vi "Write To Lights.vi"   [LabVIEW 2014]
uses:
  Common Code/Utilities/TimeManager.vi
  Common Code/Change Detect.vi
  Common Code/Change Detect Boolean.vi
  Robot Global Data.vi
types:
  T1 = typedef "Elevator Status.ctl" = cluster{"Height":dbl, "Enc Value":dbl, "Limit Override":bool, "Mode":T2, "High IR":bool, "Motor Out":dbl, "Ping Detect":bool, "Auto Elevator Indicators":T3, "Master Current":dbl, "Slave Current":dbl, "High Current":bool, "Current Tripped":bool, "Top Limit":bool, "Bottom Limit":bool, "Eject Piston":bool, "Stabilizer":bool, "Finger":bool, "Finger Height":dbl, "Finger Raw":dbl, "Finger at Bottom":bool}
  T2 = typedef "Elevator Mode.ctl" = enum16{"Manual", "Safe", "Auto"}
  T3 = typedef "Auto Elevator Indicators.ctl" = cluster{"Target Out":dbl, "Storing Trashcan?":bool, "State":T4, "In Range":bool, "Store Can Command":bool, "HP Load":bool}
  T4 = typedef "Elevator State.ctl" = enum16{"Idle", "Goto Load Position", "Wait for Load", "Load Drop", "Load Lift", "Drop Stack", "Goto Eject Position", "Eject ", "Raise Trashcan", "Open Stabilizer", "Untip Drop", "Untip Wait", "Untip Lift", "Abort Load", "HP Load Wait", "HP Load Drop", "HP Load Lift", "HP Load Abort", "Close Stabilizer", "HP Load Unfinish", "HP Load Score", "HP Load Finish", "HP Goto Finish Down", "HP Goto Finish Up", "Full"}
  T5 = typedef "WPI_DriverStationRobotMode2.ctl" = enum16{"Autonomous Disabled", "Autonomous Enabled", "Teleop Disabled", "Teleop Enabled", "Disconnected", "Finish", "Test Disabled", "Test Enabled", "Emergency Stopped"}
  T6 = typedef "WPI_DriverStationAllianceInfo.ctl" = enum16{"Red", "Blue", "Invalid"}
  T7 = typedef "Dashboard Control Data.ctl" = cluster{"Cam Exposure":dbl, "Go to angle":dbl, "Steer PID Gains":cluster{"proportional gain (Kc)":dbl, "integral time (Ti, min)":dbl, "derivative time (Td, min)":dbl}, "Steer PID output Range":cluster{"output high":dbl, "output low":dbl}, "Pressure m \nValue":dbl, "Pressure b \nValue":dbl, "Roller Command Cluster ":T8, "Elevator":T9, "Encoder Control":T11, "Auton Settings":cluster{"Drive Dist Window Size":dbl}, "Drivetrain Settings":T12, "Lance":T13}
  T8 = typedef "Roller Control.ctl" = cluster{"Intake Speed":dbl, "Turn In Speed":dbl, "Unload Speed":dbl, "Turn Out Speed":dbl, "Ping Align Tolerance":dbl, "Tote Range Threshold":dbl, "Right Pot 0":dbl, "Pot Threshold":dbl, "Left Pot 0":dbl, "Right Pot Scale":dbl, "Left Pot Scale":dbl, "Min Elevator Height":dbl, "Eject Time":dbl, "Eject US Threshold":dbl, "Anti-Twitch Time":u32, "Ping Caring Threshold":dbl, "Pot Diff Threshold":dbl, "Pinch Sustain":u32, "Absorb Give Up Threshold":dbl, "Untip In Threshold":dbl, "Untip Grab Range":dbl, "Ultrasonic Hold Time":u32, "Landscape Absorb Time":u32, "Pot Use Wait Time":u32, "Can Turn Stop Range":dbl, "HP Load Speed":dbl, "Stick Multiplier":dbl}
  T9 = typedef "Elevator DB Control.ctl" = cluster{"PID Output Range":cluster{"output high":dbl, "output low":dbl}, "PID gains":cluster{"proportional gain (Kc)":dbl, "integral time (Ti, min)":dbl, "derivative time (Td, min)":dbl}, "Height Tolerance":sgl, " Encoder Constant":dbl, "Eject Time":sgl, "Zeroing Speed":sgl, "Presets":T10, "Ping Detect Threshold":sgl, "Trashcan Detect Threshold":sgl, "Zero Filter Time":dbl, "Stabilizer Open Time":dbl, "Zero Creep Speed":dbl, "Max Current":dbl, "Current Trip Time":dbl, "Abort Pitch":dbl, "Finger m":dbl, "Finger b":dbl, "Finger max ":dbl, "Finger Stabilizer":dbl, "Finger Store":dbl, "Finger Stop Store":dbl, "Stabilizer Close Time":dbl, "Finger min":dbl, "Unstick gain":dbl, "Full Detect Max":dbl}
  T10 = typedef "Elevator Presets.ctl" = cluster{"Pickup 2 w/ Tote":sgl, "Pickup 2 w/ Trashcan":sgl, "Pickup 3 w/ Tote":sgl, "Pickup 3 w/ Trashcan":sgl, "Bottom":sgl, "Pickup 1 w/ Tote":sgl, "Pickup Trashcan":sgl, "Pickup 1 w/ Trashcan":sgl, "Eject":sgl, "Hold Low":sgl, "Step add height":sgl, "Untip Lift":dbl, "Drop Stack":dbl, "HP Load Hold":dbl, "HP Load Drop":dbl, "HP Load Hold Can":dbl, "Store can max":dbl, "HP Drag Score":dbl, "HP Drag Finish":dbl, "Finger trashcan avoid":dbl, "Full":dbl}
  T11 = typedef "Encoder Control.ctl" = cluster{"Left Tick Constant":dbl, "Right Tick Constant":dbl, "Center Tick Constant":dbl, "Reset?":bool, "Y Dist":cluster{"PID gains":cluster{"proportional gain (Kc)":dbl, "integral time (Ti, min)":dbl, "derivative time (Td, min)":dbl}}, "X Dist":cluster{"PID gains":cluster{"proportional gain (Kc)":dbl, "integral time (Ti, min)":dbl, "derivative time (Td, min)":dbl}}, "Y Stop Thresh":dbl, "Y Stop Speed":dbl, "X Stop Thresh":dbl, "X Stop Speed":dbl}
  T12 = typedef "Drivetrain Settings.ctl" = cluster{"Gyro Tolerance":sgl, "Strafe Correct max steer":sgl, "Strafe Timer Wait":sgl, "Throttle Ramp (ms)":sgl, "Strafe Ramp (ms)":sgl, "Angular rate compensation":bool, "Throttle to Rate Scale":sgl, "Rate compensation gain":sgl, "Creep Steer":sgl, "Creep Throttle":sgl}
  T13 = typedef "Pike DB Controls.ctl" = cluster{"Down Speed":dbl, "Up Speed":dbl, "Max Down Time":dbl, "Max Up Time":dbl, "Current Limit":dbl}
  T14 = typedef "WPI_AOChannelDevRef.ctl" = cluster{"DevStatus":errorcluster, "Controller":T15, "AO Channel":T16}
  T15 = typedef "FPGA_TypedefAnalogModule.ctl" = enum16{"Controller 1"}
  T16 = typedef "WPI_AnalogOutputChannel.ctl" = enum8{"AO MXP 0", "AO MXP 1", "Invalid"}
  T17 = typedef "WPI_DigitalOutputDevRef.ctl" = cluster{"Controller":T18, "DIO Channel":T19, "DevStatus":errorcluster}
  T18 = typedef "FPGA_TypedefDigitalModule.ctl" = enum16{"Controller 1"}
  T19 = typedef "FPGA_DIOChannel.ctl" = enum8{"DIO 0", "DIO 1", "DIO 2", "DIO 3", "DIO 4", "DIO 5", "DIO 6", "DIO 7", "DIO 8", "DIO 9", "DIO MXP 0", "DIO MXP 1", "DIO MXP 2", "DIO MXP 3", "DIO MXP 4", "DIO MXP 5", "DIO MXP 6", "DIO MXP 7", "DIO MXP 8", "DIO MXP 9", "DIO MXP 10", "DIO MXP 11", "DIO MXP 12", "DIO MXP 13", "DIO MXP 14", "DIO MXP 15", "Invalid"}
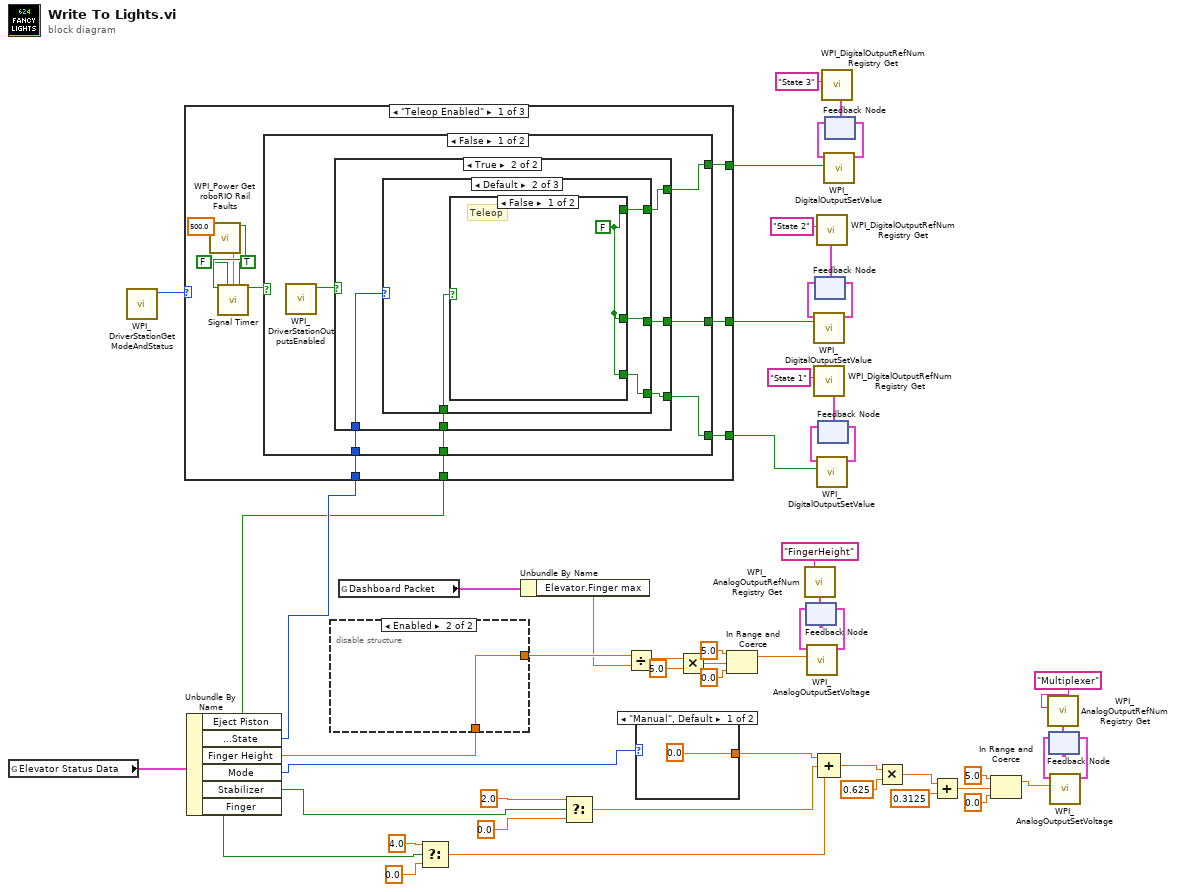
[diagram p0: block diagram]
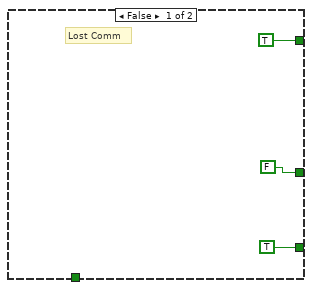
[diagram p2: hidden frame]
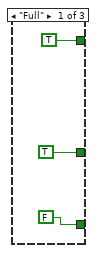
[diagram p3: hidden frame]
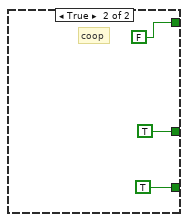
[diagram p4: hidden frame]
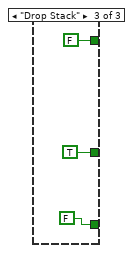
[diagram p5: hidden frame]
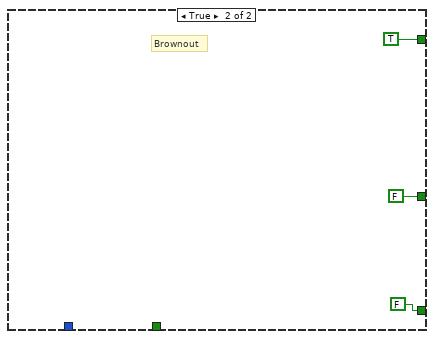
[diagram p6: hidden frame]
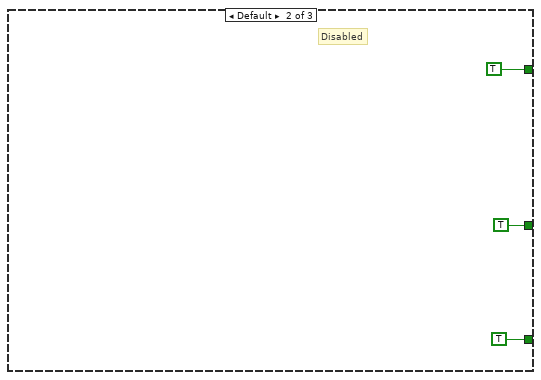
[diagram p7: hidden frame]
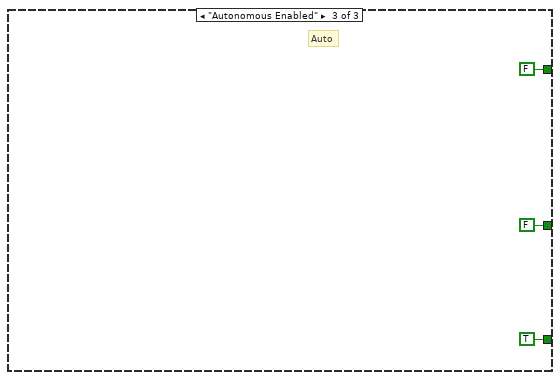
[diagram p8: hidden frame]
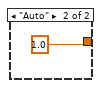
[diagram p9: hidden frame]
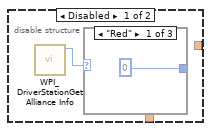
[diagram p10: hidden frame]
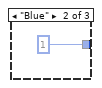
[diagram p11: hidden frame]
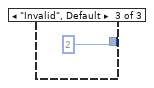
[diagram p12: hidden frame]
diagram:
  n1 = global read "Robot Global Data.vi" "Elevator Status Data"() -> (w43:T1)
  n2 = call <vilib>:"WPI_DriverStationGetModeAndStatus.vi"() -> ("Robot Mode"=w6:T5)  [unwired: 10 in, 1 out]
  n3 = Unbundle By Name(w43) -> ("Eject Piston"=w1:bool, "Auto Elevator Indicators.State"=w2:T4, "Finger Height"=w40:dbl, "Mode"=w38:T2, "Stabilizer"=w39:bool, "Finger"=w35:bool)
  n4 = case shown="\"Teleop Enabled\"" w6 {
    tunnel: [w65 TRUE FALSE] -> w5
    tunnel: [w64 TRUE FALSE] -> w4
    tunnel: [w63 TRUE TRUE] -> w3
    tunnel: w2 -> [w62 _ _]
    tunnel: w1 -> [w61 _ _]
    frame "Teleop Enabled" {
      n5 = call <vilib>:"WPI_Power Get roboRIO Rail Faults.vi"() -> ("Input Voltage Brown Out"=w60:bool)  [unwired: 11 in, 4 out]
      n6 = call "Signal Timer.vi"("Input"=w60, "Edge"=FALSE, "Interval"=500.0, "Pull"=TRUE) -> ("Filtered Output"=w56:bool)  [unwired: 11 in]
      n7 = case shown="False" w56 {
        tunnel: [w68 TRUE] -> w65
        tunnel: [w69 FALSE] -> w64
        tunnel: [w70 FALSE] -> w63
        tunnel: w62 -> [w67 _]
        tunnel: w61 -> [w66 _]
        frame False {
          n8 = call <vilib>:"WPI_DriverStationOutputsEnabled.vi"() -> ("OutputsEnabled?"=w71:bool)  [unwired: 10 in, 1 out]
          n9 = case shown="True" w71 {
            tunnel: [TRUE w76] -> w70
            tunnel: [FALSE w77] -> w69
            tunnel: [TRUE w78] -> w68
            tunnel: w67 -> [_ w79]
            tunnel: w66 -> [_ w75]
            frame False {
              # "Lost Comm"
            }
            frame True {
              n10 = case shown="Default" w79 {
                tunnel: [TRUE w86 FALSE] -> w78
                tunnel: [TRUE w84 TRUE] -> w77
                tunnel: [FALSE w85 FALSE] -> w76
                tunnel: w75 -> [_ w83 _]
                frame "Full" {
                }
                frame Default {
                  n11 = case shown="False" w83 {
                    tunnel: [w87 FALSE] -> w86
                    tunnel: [w87 TRUE] -> w85
                    tunnel: [w87 TRUE] -> w84
                    frame False {
                      w87 = FALSE
                      # "Teleop"
                    }
                    frame True {
                      # "coop"
                    }
                  }
                }
                frame "Drop Stack" {
                }
              }
            }
          }
        }
        frame True {
          # "Brownout"
        }
      }
    }
    frame Default {
      # "Disabled"
    }
    frame "Autonomous Enabled" {
      # "Auto"
    }
  }
  n12 = disable-structure shown="Enabled" {
    disable-tunnel: w40 -> [_ w107]
    disable-tunnel: [_ w107] -> w29
    frame Disabled {
      n13 = call <vilib>:"WPI_DriverStationGet Alliance Info.vi"() -> ("Alliance"=w103:T6)  [unwired: 10 in, 1 out]
      n14 = case shown="\"Red\"" w103 {
        tunnel: [u8 0 u8 1 u8 2 ("I2CRegister")] -> _
        frame "Red" {
        }
        frame "Blue" {
        }
        frame "Invalid", Default {
        }
      }
    }
    frame Enabled {
    }
  }
  n15 = global read "Robot Global Data.vi" "Dashboard Packet"() -> (w30:T7)
  n16 = Select(t=sgl 4.0 ("unsigned 8bit integer"), s=w35, f=sgl 0.0 ("unsigned 8bit integer")) -> (s? t:f=w19:sgl)
  n17 = Unbundle By Name(w30) -> ("Elevator.Finger max"=w28:dbl)
  n18 = Select(t=sgl 2.0 ("unsigned 8bit integer"), s=w39, f=sgl 0.0 ("unsigned 8bit integer")) -> (s? t:f=w20:sgl)
  n19 = Divide(x=w29, y=w28) -> (x/y=w27:dbl)
  n20 = case shown="\"Manual\", Default" w38 {
    tunnel: [sgl 0.0 sgl 1.0 ("I2CRegister")] -> w21
    frame "Manual", Default {
    }
    frame "Auto" {
    }
  }
  n21 = Multiply(x=w27, y=5.0) -> (x*y=w25:dbl)
  n22 = In Range and Coerce(upper limit=5.0, x=w25, lower limit=0.0) -> (coerced(x)=w22:dbl)  [unwired: 1 out]
  n23 = call <vilib>:"WPI_AnalogOutputRefNum Registry Get.vi"("refnum name"="FingerHeight") -> ("AODeviceRef"=w33:T14)  [unwired: 9 in, 1 out]
  n24 = feedback #1(w33) -> (w32:T14)
  n25 = call <vilib>:"WPI_AnalogOutputSetVoltage.vi"("Voltage"=w22, "AODeviceRef"=w32) -> ("AODeviceRef"=w31:T14)  [unwired: 8 in, 1 out]
  n26 = feedback-in #1(w31) -> ()
  n27 = call <vilib>:"WPI_DigitalOutputRefNum Registry Get.vi"("refnum name"="State 1") -> ("DigitalOutputDevRef"=w54:T17)  [unwired: 9 in, 1 out]
  n28 = call <vilib>:"WPI_DigitalOutputRefNum Registry Get.vi"("refnum name"="State 2") -> ("DigitalOutputDevRef"=w48:T17)  [unwired: 9 in, 1 out]
  n29 = feedback #2(w48) -> (w50:T17)
  n30 = call <vilib>:"WPI_DigitalOutputSetValue.vi"("Value"=w4, "DigitalOutputDevRef"=w50) -> ("DigitalOutputDevRef"=w49:T17)  [unwired: 8 in, 1 out]
  n31 = feedback-in #2(w49) -> ()
  n32 = feedback #3(w54) -> (w52:T17)
  n33 = call <vilib>:"WPI_DigitalOutputSetValue.vi"("Value"=w3, "DigitalOutputDevRef"=w52) -> ("DigitalOutputDevRef"=w53:T17)  [unwired: 8 in, 1 out]
  n34 = feedback-in #3(w53) -> ()
  n35 = Compound Arithmetic op=ADD(w21, w20, w19) -> (w18:sgl)
  n36 = call <vilib>:"WPI_DigitalOutputRefNum Registry Get.vi"("refnum name"="State 3") -> ("DigitalOutputDevRef"=w47:T17)  [unwired: 9 in, 1 out]
  n37 = feedback #4(w47) -> (w46:T17)
  n38 = call <vilib>:"WPI_DigitalOutputSetValue.vi"("Value"=w5, "DigitalOutputDevRef"=w46) -> ("DigitalOutputDevRef"=w44:T17)  [unwired: 8 in, 1 out]
  n39 = feedback-in #4(w44) -> ()
  n40 = Multiply(x=w18, y=sgl 0.625) -> (x*y=w16:sgl)
  n41 = Add(x=w16, y=sgl 0.3125) -> (x+y=w10:sgl)
  n42 = In Range and Coerce(upper limit=5.0, x=w10, lower limit=0.0) -> (coerced(x)=w9:dbl)  [unwired: 1 out]
  n43 = call <vilib>:"WPI_AnalogOutputRefNum Registry Get.vi"("refnum name"="Multiplexer") -> ("AODeviceRef"=w13:T14)  [unwired: 9 in, 1 out]
  n44 = feedback #5(w13) -> (w8:T14)
  n45 = call <vilib>:"WPI_AnalogOutputSetVoltage.vi"("Voltage"=w9, "AODeviceRef"=w8) -> ("AODeviceRef"=w14:T14)  [unwired: 8 in, 1 out]
  n46 = feedback-in #5(w14) -> ()
